vi "daq_z_scan_threshold.vi"(0 "channels in":refnum<k21>, 5 "N":i32, 7 "lower threshold":dbl, 9 "upper threshold":dbl, 11 "error in":errorcluster) -> (4 "task out":refnum<k21>, 6 "OA":dbl[][](array[numeric]), 8 "CA":dbl[][](array[numeric]), 10 "REF":dbl[][](array[numeric]), 15 "error out":errorcluster)   [LabVIEW 2010]
uses:
  <vilib>/DAQmx/read.llb/DAQmx Read (Analog 2D DBL NChan NSamp).vi
  <vilib>/Analysis/NI_AALBase.lvlib
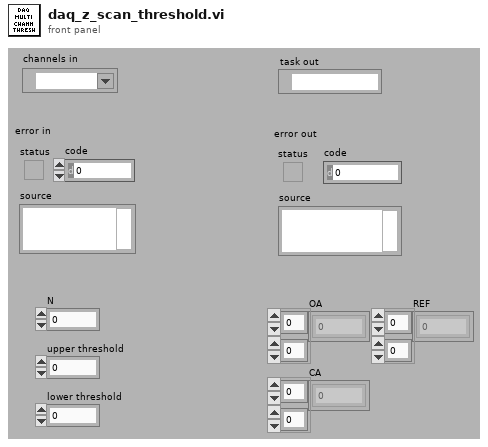
[diagram p1: front panel]
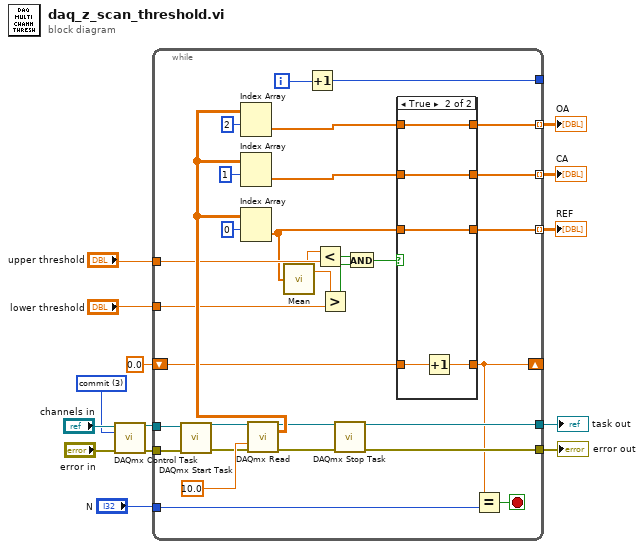
[diagram p0: block diagram]
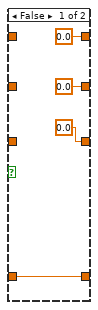
[diagram p2: hidden frame]
diagram:
  w12 = 3 items=["verify"=2, "reserve"=4, "commit"=3, "unreserve"=5, "abort"=6] ("action")
  n1 = call <vilib>:"DAQmx Control Task.vi"("task/channels in"="channels in", "action"=w12, "error in"="error in") -> ("task out"=w11:refnum<k21>, "error out"=w10:errorcluster)  [unwired: 11 in]
  n2 = while {
    tunnel: w11 -> [w40]
    tunnel: w10 -> [w39]
    tunnel: [w34] -> w9
    tunnel: [w33] -> w8
    tunnel: [w31] -> w3 mode=indexing
    tunnel: [w30] -> w2 mode=indexing
    tunnel: [w29] -> w1 mode=indexing
    shift-right: [w26] -> _
    shift-left: 0.0 -> [w28]
    tunnel: "N" -> [w27]
    tunnel: [w23] -> _
    tunnel: "upper threshold" -> [w22]
    tunnel: "lower threshold" -> [w17]
    i -> [w24]
    stop <- w25 stop-if-true
    n3 = call <vilib>:"DAQmx Start Task.vi"("task/channels in"=w40, "error in"=w39) -> ("task out"=w38:refnum<k21>, "error out"=w37:errorcluster)  [unwired: 12 in]
    n4 = call-poly <vilib>:"DAQmx Read.vi"("task/channels in"=w38, "timeout"=10.0, "error in"=w37) -> ("task out"=w36:refnum<k21>, "data"=w41:dbl[][], "error out"=w35:errorcluster)  [unwired: 10 in]
    n5 = Index Array(array=w41, index (row)=2 ("index")) -> (element=w20:dbl[])  [unwired: 1 in]
    n6 = Index Array(array=w41, index (row)=1 ("index")) -> (element=w32:dbl[])  [unwired: 1 in]
    n7 = Index Array(array=w41, index (row)=0 ("index")) -> (element=w16:dbl[])  [unwired: 1 in]
    n8 = call <vilib>:"Mean.vi"("X"=w16) -> ("mean"=w15:dbl)  [unwired: 1 out]
    n9 = Increment(x=w24) -> (x+1=w23:i32)
    n10 = Less?(x=w15, y=w22) -> (x < y?=w21:bool)
    n11 = Greater?(x=w15, y=w17) -> (0:w19:bool)
    n12 = call <vilib>:"DAQmx Stop Task.vi"("task/channels in"=w36, "error in"=w35) -> ("task out"=w34:refnum<k21>, "error out"=w33:errorcluster)  [unwired: 12 in]
    n13 = And(x=w21, y=w19) -> (x .and. y?=w18:bool)
    n14 = case shown="True" w18 {
      tunnel: w20 -> [_ w54]
      tunnel: w32 -> [_ w53]
      tunnel: w16 -> [_ w52]
      tunnel: [0.0 ("Waveform") w54] -> w31
      tunnel: [0.0 ("Waveform") w53] -> w30
      tunnel: [0.0 ("Waveform") w52] -> w29
      tunnel: [w46 w51] -> w26
      tunnel: w28 -> [w46 w50]
      frame False {
      }
      frame True {
        n15 = Increment(x=w50) -> (x+1=w51:dbl)
      }
    }
    n16 = Equal?(x=w26, y=w27) -> (x = y?=w25:bool)
  }
  "error out" <- w8
  "task out" <- w9
  "OA" <- w3
  "CA" <- w2
  "REF" <- w1
